vi "frequency_3db.vi"(10 "Misure":dbl[](array[numeric]), 11 "Frequenze":dbl[](array[numeric])) -> (2 "Frequenza non trovata":bool, 3 "Frequenza -3dB":dbl)   [LabVIEW 2021]
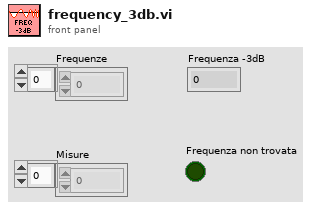
[diagram p1: front panel]
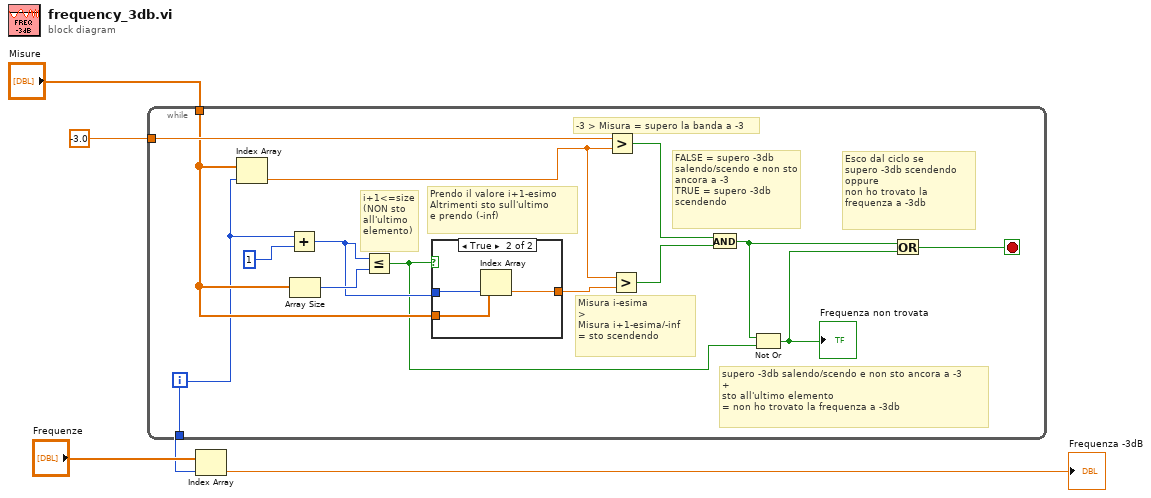
[diagram p0: block diagram]
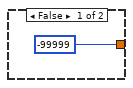
[diagram p2: hidden frame]
diagram:
  n1 = while {
    tunnel: -3.0 -> [w19]
    tunnel: "Misure" -> [w11]
    tunnel: [w10] -> w2
    i -> [w10]
    stop <- w7 stop-if-true
    # "supero -3db salendo/scendo e non sto ancora a -3\n+\nsto all'ultimo elemento\n= non ho trovato la frequenza a -3db"
    # "Esco dal ciclo se\nsupero -3db scendendo\noppure\nnon ho trovato la frequenza a -3db"
    # "FALSE = supero -3db salendo/scendo e non sto ancora a -3\nTRUE = supero -3db scendendo"
    # "Misura i-esima\n>\nMisura i+1-esima/-inf\n= sto scendendo"
    # "Prendo il valore i+1-esimo\nAltrimenti sto sull'ultimo\ne prendo (-inf)"
    # "i+1<=size\n(NON sto\nall'ultimo\nelemento)"
    # "-3 > Misura = supero la banda a -3"
    n2 = Index Array(array=w11, index=w10) -> (element=w13:dbl)
    n3 = Add(x=w10, y=1) -> (x+y=w16:i32)
    n4 = Array Size(array=w11) -> (size(s)=w17:i32)
    n5 = Less Or Equal?(x=w16, y=w17) -> (x <= y?=w9:bool)
    n6 = case shown="True" w9 {
      tunnel: w11 -> [_ w23]
      tunnel: w16 -> [_ w22]
      tunnel: [-99999 w21] -> w14
      frame False {
      }
      frame True {
        n7 = Index Array(array=w23, index=w22) -> (element=w21:dbl)
      }
    }
    n8 = Greater?(x=w19, y=w13) -> (0:w15:bool)
    n9 = Greater?(x=w13, y=w14) -> (0:w12:bool)
    n10 = And(x=w15, y=w12) -> (x .and. y?=w8:bool)
    n11 = Not Or(1:w9, 2:w8) -> (0:w6:bool)
    "Frequenza non trovata" <- w6
    n12 = Or(x=w8, y=w6) -> (x .or. y?=w7:bool)
  }
  n13 = Index Array(array="Frequenze", index=w2) -> (element=→"Frequenza -3dB":dbl)
